vi "testV6-Graph.vi"() -> ()   [LabVIEW 2020]
uses:
  <vilib>/DAQmx/read.llb/DAQmx Read (Analog 2D DBL NChan NSamp).vi
  <vilib>/Analysis/baseanly.llb/Mean (DBL).vi
  <vilib>/DAQmx/miscellaneous.llb/DAQmx Fill In Error Info.vi
  <vilib>/Analysis/NI_AALBase.lvlib
  <resource>/objmgr/daqmx.rc
panel:
  out "element":dbl
  out "?":timestamp
  out "Channels":refnum<k21>[](array[refnum])
  in  "stop":bool
  out "size(s)":i32
  out "NumDevices":u32
  out "x/y":dbl
  in  "?":T1(tab)
  in  "Next Button":bool
  in  "Stop Button 2":bool
  out "Graph Running":bool
  in  "Resolution":u8 min=10
  in  "Select Channel":u8
  in  "Stop Button":bool
  in  "Play Button":bool
  out "Module 3":bool
  out "Module 2":bool
  out "Module 1":bool
  in  "Sampling Time":u32=5
  in  "Read Time (s)":u32=60
  out "3":bool
  out "2":bool
  out "1":bool
  in  "Running Module":u8=1 min=1 max=3
  in  "Module 3 Task":refnum<k21>="MyTemperatureTask_2"
  out "?":waveform(dbl)(graph)
  in  "Module 3 File Data Location":path=path "E:/KMUTT/Master Degree/labviewjgsee/log/Module3"
  in  "Module 2 File Data Location":path=path "E:/KMUTT/Master Degree/labviewjgsee/log/Module2"
  in  "Module 2 Task":refnum<k21>="MyTemperatureTask_1"
  in  "Module 1 File Data Location":path=path "E:/KMUTT/Master Degree/labviewjgsee/log/Module1"
  in  "Module 1 Task":refnum<k21>="MyTemperatureTask"
  in  "DAQmx Device Name":tag
  out "Table Module 1":string[][](table)
  out "Table Module 2":string[][](table)
  out "Table Module 3":string[][](table)
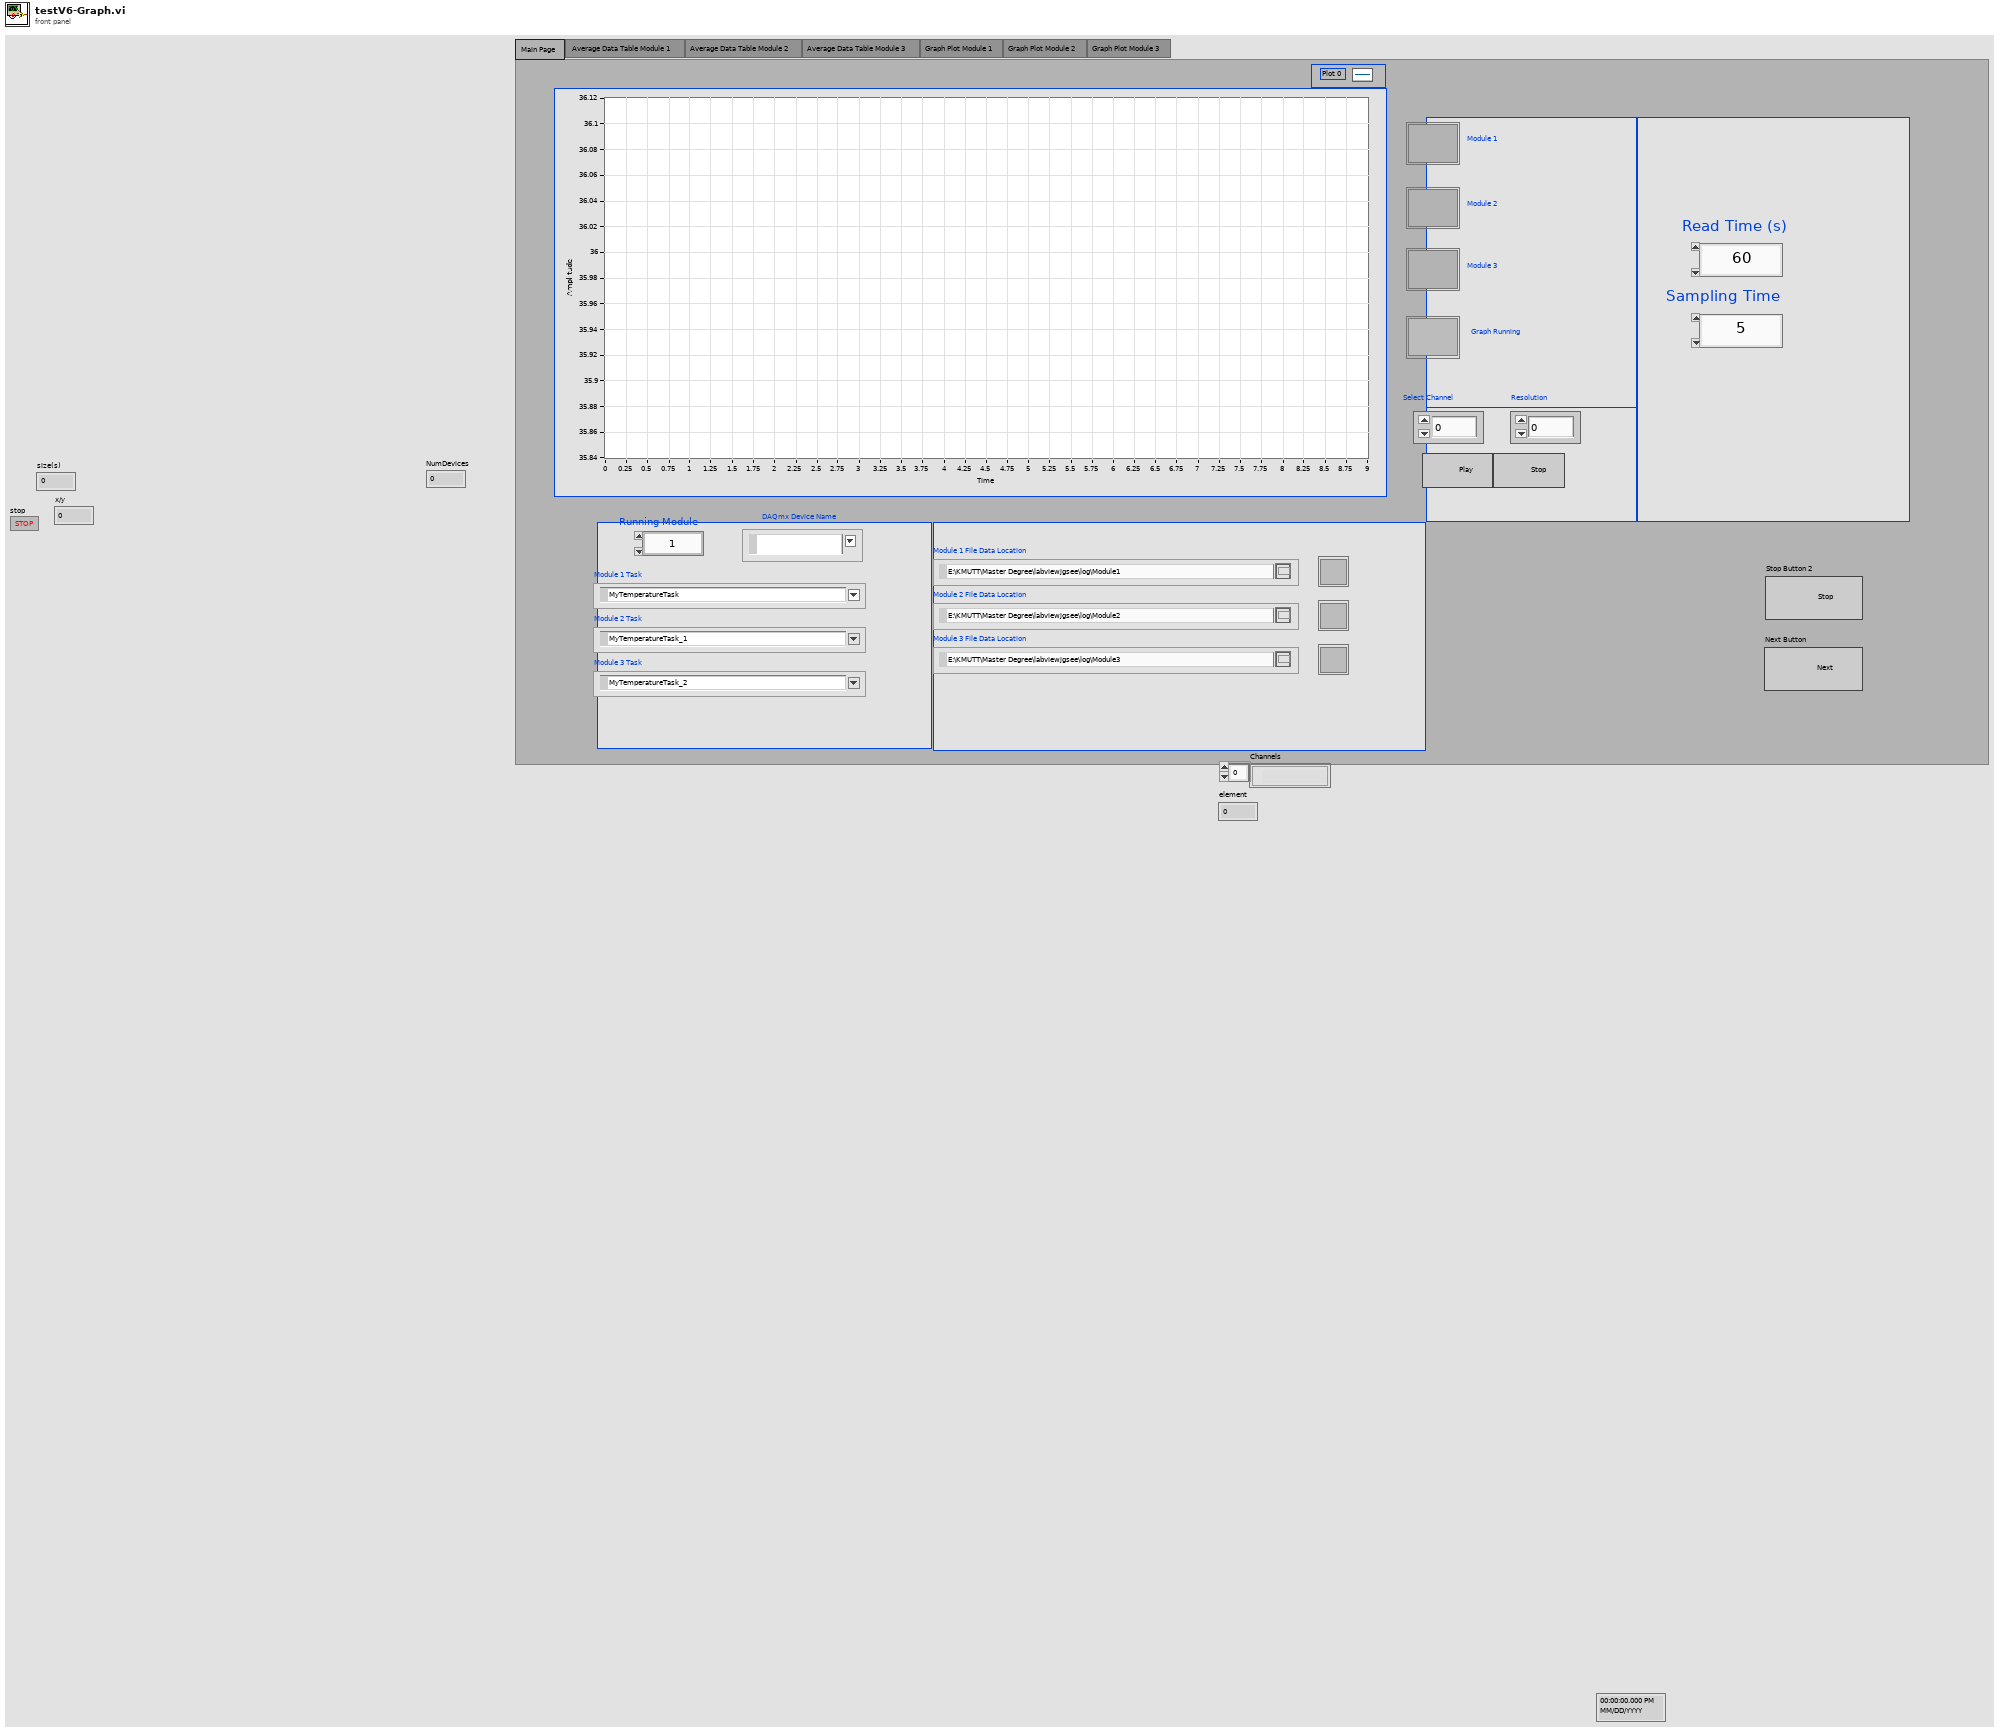
[diagram p1: front panel]
types:
  T1 = enum32{"Main Page ", " Average Data Table Module 1", "Average Data Table Module 2", "Average Data Table Module 3", "Graph Plot Module 1", "Graph Plot Module 2", "Graph Plot Module 3"}
  T2 = enum16{"open", "replace", "create", "open or create", "replace or create", "replace or create with confirmation"}
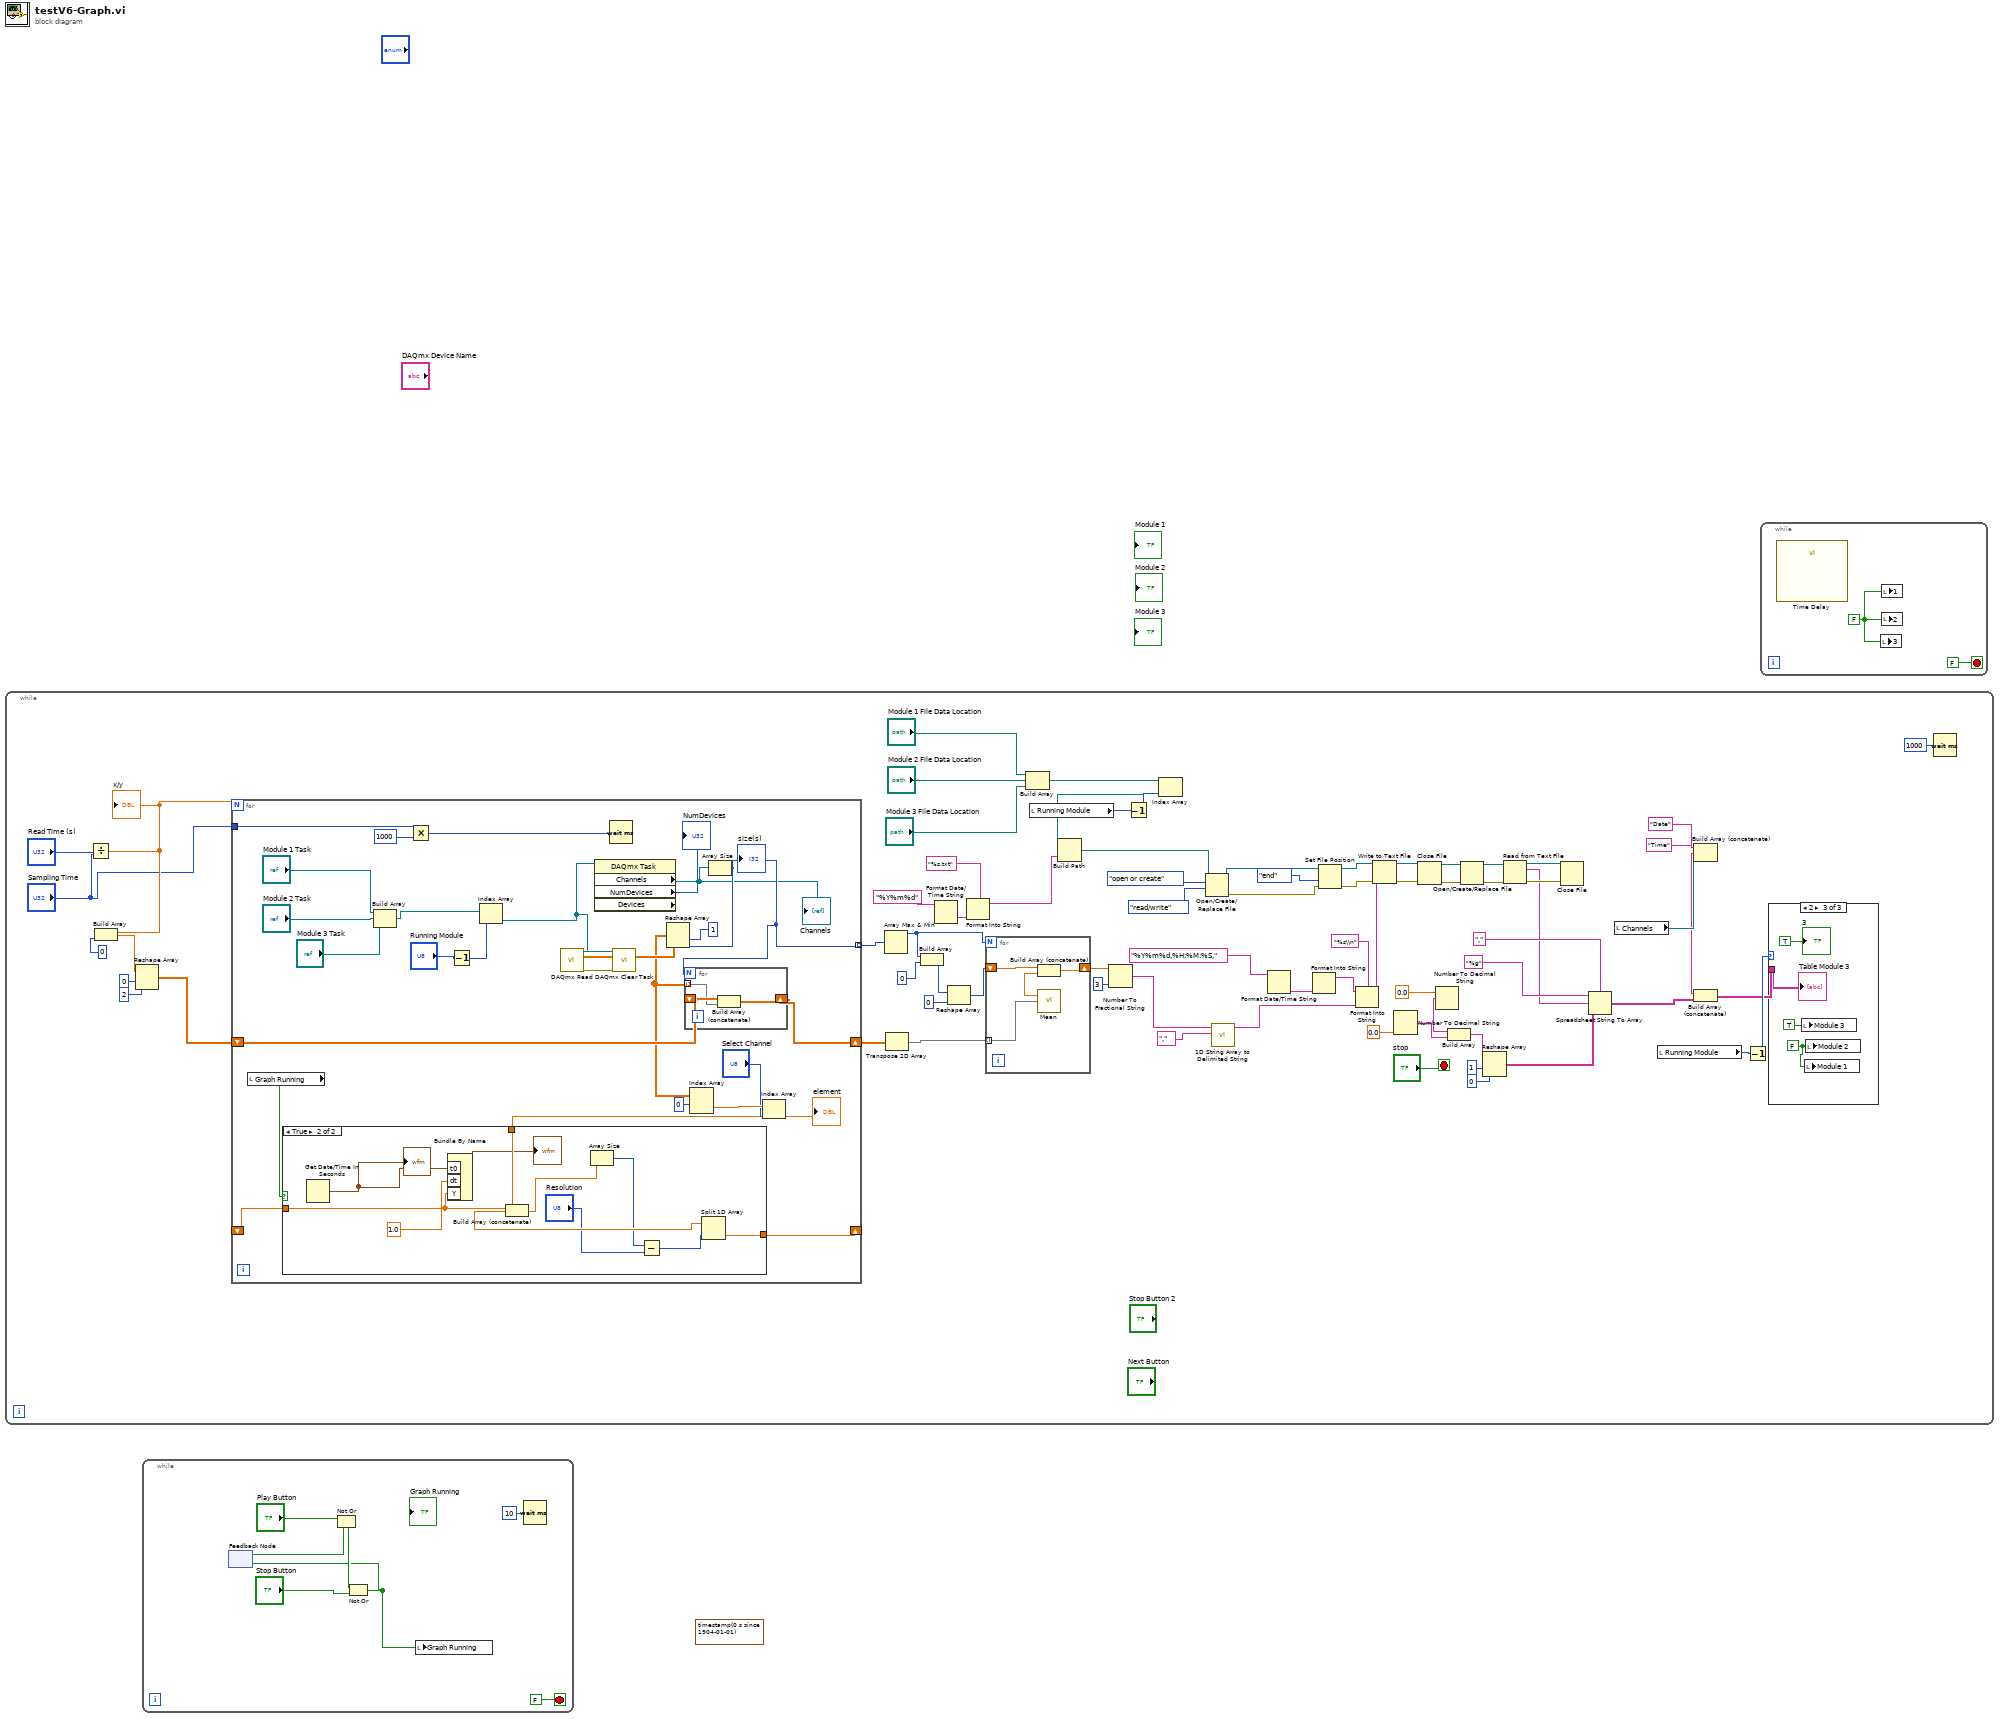
[diagram p0: block diagram]
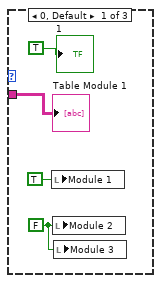
[diagram p2: hidden frame]
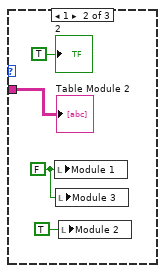
[diagram p3: hidden frame]
diagram:
  (unwired) timestamp(0 s since 1904-01-01)
  n1 = while {
    stop <- "stop" stop-if-true
    n2 = Divide(x="Read Time (s)", y="Sampling Time") -> (x/y=w49:dbl)
    "x/y" <- w49
    n3 = Build Array(w49, 0 ("element")) -> (w53:dbl[])
    n4 = Reshape Array(w53, 0 ("dimension size"), 2 ("dimension size")) -> (w50:dbl[][])
    n5 = for {
      N: w49 -> [_]
      shift-right: [w110] -> w18
      shift-left: w50 -> [w109]
      tunnel: "Sampling Time" -> [w108]
      tunnel: [w106] -> w48 mode=indexing
      shift-right: [w89] -> _
      shift-left: _ -> [w88]
      n6 = local read "Graph Running"() -> (w87:bool)
      n7 = Build Array("Module 1 Task", "Module 2 Task", "Module 3 Task") -> (w101:refnum<k21>[])
      n8 = Multiply(x=w108, y=u32 1000) -> (x*y=w96:u32)
      n9 = Decrement(x="Running Module") -> (x-1=w97:u8)
      n10 = Index Array(array=w101, index=w97) -> (element=w100:refnum<k21>)
      n11 = call-poly <vilib>:"DAQmx Read.vi"("task/channels in"=w100) -> ("task out"=w112:refnum<k21>, "data"=w105:dbl[][], "error out"=w113:errorcluster)  [unwired: 12 in]
      n12 = property class="DAQmx Task" props=["Channels", "NumDevices", "Devices"](reference=w100) -> ("Channels"=w95:refnum<k21>[], "NumDevices"=→"NumDevices":u32)  [unwired: 1 in, 3 out]
      "Channels" <- w95
      n13 = Wait (ms)(milliseconds to wait=w96) -> ()  [unwired: 1 out]
      n14 = call <vilib>:"DAQmx Clear Task.vi"("task in"=w112, "error in"=w113) -> ()  [unwired: 13 in, 1 out]
      n15 = Array Size(array=w95) -> (size(s)=w106:i32)
      "size(s)" <- w106
      n16 = Reshape Array(w105, 1 ("dimension size"), w106) -> (w94:dbl[][])
      n17 = for {
        N: w106 -> [_]
        shift-right: [w125] -> w110
        shift-left: w109 -> [w126]
        tunnel: w94 -> [w124] mode=indexing
        n18 = Build Array (concatenate)(w126, w124) -> (w125:dbl[][])
      }
      n19 = Index Array(array=w94, index (row)=0) -> (element=w92:dbl[])  [unwired: 1 in]
      n20 = Index Array(array=w92, index="Select Channel") -> (element=w90:dbl)
      "element" <- w90
      n21 = case shown="True" w87 {
        tunnel: w90 -> [_ w121]
        tunnel: [_ w118] -> w89
        tunnel: w88 -> [_ w117]
        frame False {
        }
        frame True {
          n22 = Get Date/Time In Seconds() -> (seconds since 1Jan1904=w123:timestamp)
          "?" <- w123
          n23 = Bundle By Name("t0"=w123, "dt"=1.0, "Y"=w117) -> (→"?":waveform(dbl))  [unwired: 1 in]
          n24 = Build Array (concatenate)(w117, w121) -> (w119:dbl[])
          n25 = Array Size(array=w119) -> (size(s)=w115:i32)
          n26 = Subtract(x=w115, y="Resolution") -> (x-y=w116:i32)
          n27 = Split 1D Array(array=w119, index=w116) -> (second subarray=w118:dbl[])  [unwired: 1 out]
        }
      }
    }
    n28 = Array Max & Min(array=w48) -> (max value=w45:i32)  [unwired: 3 out]
    n29 = Transpose 2D Array(2D array=w18) -> (transposed array=w47:dbl[][])
    n30 = Build Array(w45, 0 ("element")) -> (w43:i32[])
    n31 = Format Date/Time String(time format string (%c)="%Y%m%d") -> (date/time string=w65:string)  [unwired: 2 in]
    n32 = Reshape Array(w43, 0 ("dimension size")) -> (w42:i32[])
    n33 = Format Into String(format string="%s.txt", w65) -> (resulting string=w63:string)  [unwired: 2 in, 1 out]
    n34 = for {
      N: w45 -> [_]
      tunnel: w47 -> [w130] mode=indexing
      shift-right: [w128] -> w55
      shift-left: w42 -> [w127]
      n35 = call-poly <vilib>:"Mean.vi"("X"=w130) -> ("mean"=w129:dbl)  [unwired: 1 out]
      n36 = Build Array (concatenate)(w127, w129) -> (w128:dbl[])
    }
    n37 = Build Array("Module 1 File Data Location", "Module 2 File Data Location", "Module 3 File Data Location") -> (w11:path[])
    n38 = local read "Running Module"() -> (w12:u8)
    n39 = Number To Fractional String(number=w55, precision (6)=i16 3) -> (F-format string=w56:string[])  [unwired: 2 in]
    n40 = Decrement(x=w12) -> (x-1=w10:u8)
    n41 = Index Array(array=w11, index=w10) -> (element=w9:path)
    n42 = Build Path(base path=w9, name or relative path=w63) -> (appended path=w62:path)
    n43 = Open/Create/Replace File(file path (use dialog)=w62, operation (0:open)=T2."open or create", access (0:read/write)=enum16{"read/write", "read-only", "write-only"}."read/write") -> (refnum out=w40:refnum<file>, error out=w69:errorcluster)  [unwired: 3 in, 1 out]
    n44 = call <vilib>:"1D String Array to Delimited String.vi"("delimiter"="," ("format string"), "string array"=w56) -> ("delimited string"=w61:string)  [unwired: 9 in]
    n45 = Format Date/Time String(time format string (%c)="%Y%m%d,%H:%M:%S,") -> (date/time string=w58:string)  [unwired: 2 in]
    n46 = Format Into String(w58) -> (resulting string=w57:string)  [unwired: 3 in, 1 out]
    n47 = Set File Position(refnum=w40, from (0:start)=enum16{"start", "end", "current"}."end", error in=w69) -> (refnum out=w70:refnum<file>, error out=w68:errorcluster)  [unwired: 1 in]
    n48 = Format Into String(format string="%s\\n", initial string=w57, w61) -> (resulting string=w32:string)  [unwired: 1 in, 1 out]
    n49 = Write to Text File(file (use dialog)=w70, text=w32, error in=w68) -> (refnum out=w39:refnum<file>, error out=w38:errorcluster)  [unwired: 1 in, 1 out]
    n50 = Number To Decimal String(number=0.0 ("element")) -> (decimal integer string=w20:string)  [unwired: 1 in]
    n51 = Close File(refnum=w39, error in=w38) -> (path=w37:path, error out=w36:errorcluster)
    n52 = Number To Decimal String(number=0.0 ("element")) -> (decimal integer string=w22:string)  [unwired: 1 in]
    n53 = Build Array(w22, w20) -> (w24:string[])
    n54 = Open/Create/Replace File(file path (use dialog)=w37, error in=w36) -> (refnum out=w35:refnum<file>, error out=w34:errorcluster)  [unwired: 4 in, 1 out]
    n55 = Reshape Array(w24, 1 ("dimension size"), 0 ("dimension size")) -> (w25:string[][])
    n56 = Read from Text File(file (use dialog)=w35, error in=w34) -> (refnum out=w33:refnum<file>, text=w28:string, error out=w29:errorcluster)  [unwired: 2 in, 1 out]
    n57 = Close File(refnum=w33, error in=w29) -> ()  [unwired: 2 out]
    n58 = Spreadsheet String To Array(delimiter (Tab)=",", format string="%g", spreadsheet string=w28, array type (2D Dbl)=w25) -> (array=w6:string[][])
    n59 = local read "Channels"() -> (w2:refnum<k21>[])
    n60 = local read "Running Module"() -> (w8:u8)
    n61 = Build Array (concatenate)("Date", "Time", w2) -> (w1:string[])
    n62 = Build Array (concatenate)(w1, w6) -> (w5:string[][])
    n63 = Decrement(x=w8) -> (x-1=w7:u8)
    n64 = case shown="2" w7 {
      tunnel: w5 -> [w78 w82 w86]
      frame 0, Default {
        w75 = FALSE ("Module 2")
        n65 = local write "Module 1"(TRUE ("Module 1")) -> ()
        n66 = local write "Module 2"(w75) -> ()
        n67 = local write "Module 3"(w75) -> ()
        "Table Module 1" <- w78
        "1" <- TRUE ("1")
      }
      frame 1 {
        w79 = FALSE ("Module 1")
        n68 = local write "Module 1"(w79) -> ()
        n69 = local write "Module 3"(w79) -> ()
        n70 = local write "Module 2"(TRUE ("Module 2")) -> ()
        "Table Module 2" <- w82
        "2" <- TRUE ("2")
      }
      frame 2 {
        w83 = FALSE ("Module 2")
        n71 = local write "Module 3"(TRUE ("Module 3")) -> ()
        n72 = local write "Module 1"(w83) -> ()
        n73 = local write "Module 2"(w83) -> ()
        "Table Module 3" <- w86
        "3" <- TRUE ("3")
      }
    }
    n74 = Wait (ms)(milliseconds to wait=u32 1000) -> ()  [unwired: 1 out]
  }
  n75 = while {
    stop <- FALSE stop-if-true
    n76 = feedback #1() -> (w132:bool)  [unwired: 1 in]
    n77 = Not Or(1:w132, 2:"Play Button") -> (0:w133:bool)
    n78 = Not Or(1:"Stop Button", 2:w133) -> (0:w131:bool)
    n79 = feedback-in #1(w131) -> ()
    n80 = local write "Graph Running"(w131) -> ()
    n81 = Wait (ms)(milliseconds to wait=u32 10) -> ()  [unwired: 1 out]
  }
  n82 = while {
    stop <- FALSE stop-if-true
    w139 = FALSE ("1")
    n83 = call "Time Delay"() -> ()  [unwired: 11 in, 1 out]
    n84 = local write "3"(w139) -> ()
    n85 = local write "1"(w139) -> ()
    n86 = local write "2"(w139) -> ()
  }
